vi "Scripting Start.vi"(9 "B":dbl, 10 "A":dbl) -> (2 "C":dbl)   [LabVIEW 2026]
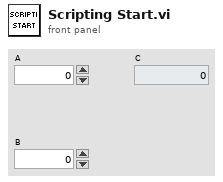
[diagram p1: front panel]
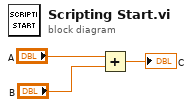
[diagram p0: block diagram]
diagram:
  n1 = Add(x="A", y="B") -> (x+y=→"C":dbl)
